vi "dzielenie.vi"() -> ()   [LabVIEW 2017]
panel:
  out "Errors":string
  out "Remainder":dbl
  out "x/y":dbl
  in  "y":dbl
  in  "x":dbl
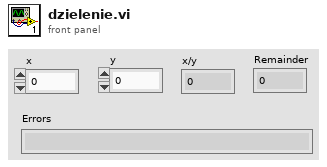
[diagram p1: front panel]
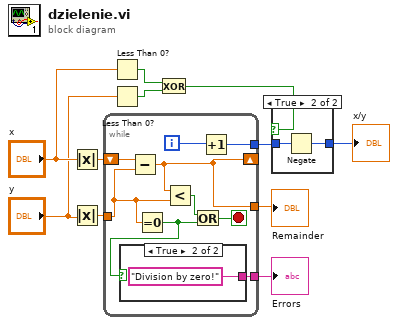
[diagram p0: block diagram]
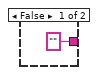
[diagram p3: hidden frame]
diagram:
  n1 = Absolute Value(x="x") -> (abs(x)=w10:dbl)
  n2 = Absolute Value(x="y") -> (abs(x)=w9:dbl)
  n3 = while {
    tunnel: w9 -> [w14]
    shift-right: [w19] -> _
    shift-left: w10 -> [w20]
    tunnel: [w19] -> w11
    tunnel: [w18] -> w8
    tunnel: [w12] -> w1
    i -> [w17]
    stop <- w15 stop-if-true
    n4 = Subtract(x=w20, y=w14) -> (x-y=w19:dbl)
    n5 = Equal To 0?(x=w14) -> (x = 0?=w13:bool)
    n6 = case shown="True" w13 {
      tunnel: ["" ("Errors") "Division by zero!" ("Errors")] -> w12
      frame False {
      }
      frame True {
      }
    }
    n7 = Less?(x=w19, y=w14) -> (x < y?=w16:bool)
    n8 = Or(x=w16, y=w13) -> (x .or. y?=w15:bool)
    n9 = Increment(x=w17) -> (x+1=w18:i32)
  }
  "Remainder" <- w11
  "Errors" <- w1
  n10 = Less Than 0?(x="x") -> (x < 0?=w4:bool)
  n11 = Less Than 0?(x="y") -> (x < 0?=w3:bool)
  n12 = Exclusive Or(1:w3, 2:w4) -> (0:w2:bool)
  n13 = case shown="True" w2 {
    tunnel: w8 -> [w23 w25]
    tunnel: [w23 w24] -> w7
    frame False {
    }
    frame True {
      n14 = Negate(x=w25) -> (-x=w24:i32)
    }
  }
  "x/y" <- w7
